vi "TrendsD01.vi"() -> ()   [LabVIEW 2019, in "D01.lvlib"]
uses:
  D01.lvlib
  <vilib>/measure/mamon.llb/Trigger Detection for 1 Channel.vi
  <vilib>/measure/NI_MAPro.lvlib
panel:
  out "No Change":bool
  out "Sudden Change":bool
  out "Decrease":bool
  out "Increase":bool
  out "Previous  ES":dbl
  out "Present  Speed":dbl
  out "Present Error":dbl format="%#.2g"
  out "Previous Error":dbl
  out "Previous  Speed":dbl
  out "Previous PW":dbl caption="Control Information"
  out "Pulse Trends":waveform(i16)[](graph) caption="Waveform Chart - Dark"
  in  "Close":bool
  out "disc name":string="Disc 01 Trends"
  out "dsgs":string="DSGS"
  out "Speed Trend":waveform(dbl)(graph) caption="Waveform Chart - Dark"
  out "Average Trend":waveform(dbl)[](graph) caption="Waveform Chart - Dark"
  out "Live Trend":waveform(dbl)[](graph) caption="Waveform Chart - Dark"
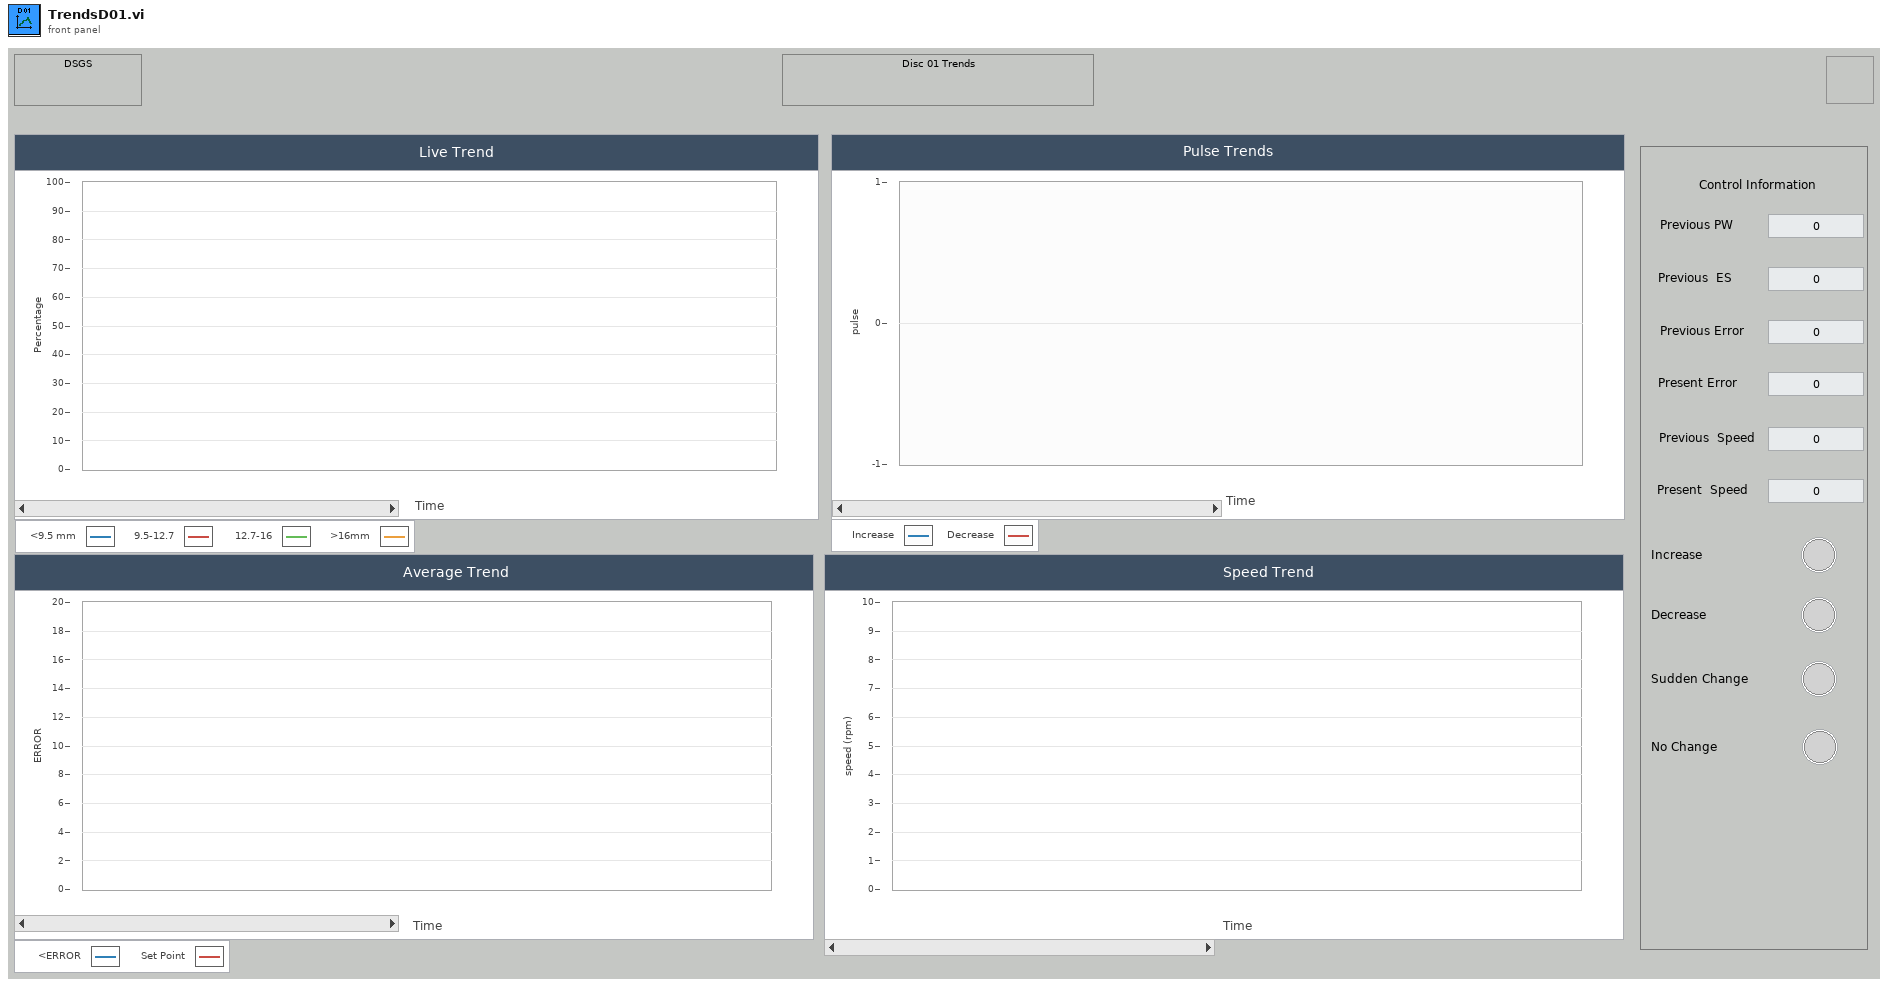
[diagram p1: front panel]
types:
  T1 = cluster{"decrease D01":bool, "increase D01":bool, "no change D01":bool, "sudden change D01":bool, "last error 01":dbl, "previous speed D01":dbl, "puls width D01":dbl, "slope D01":dbl}
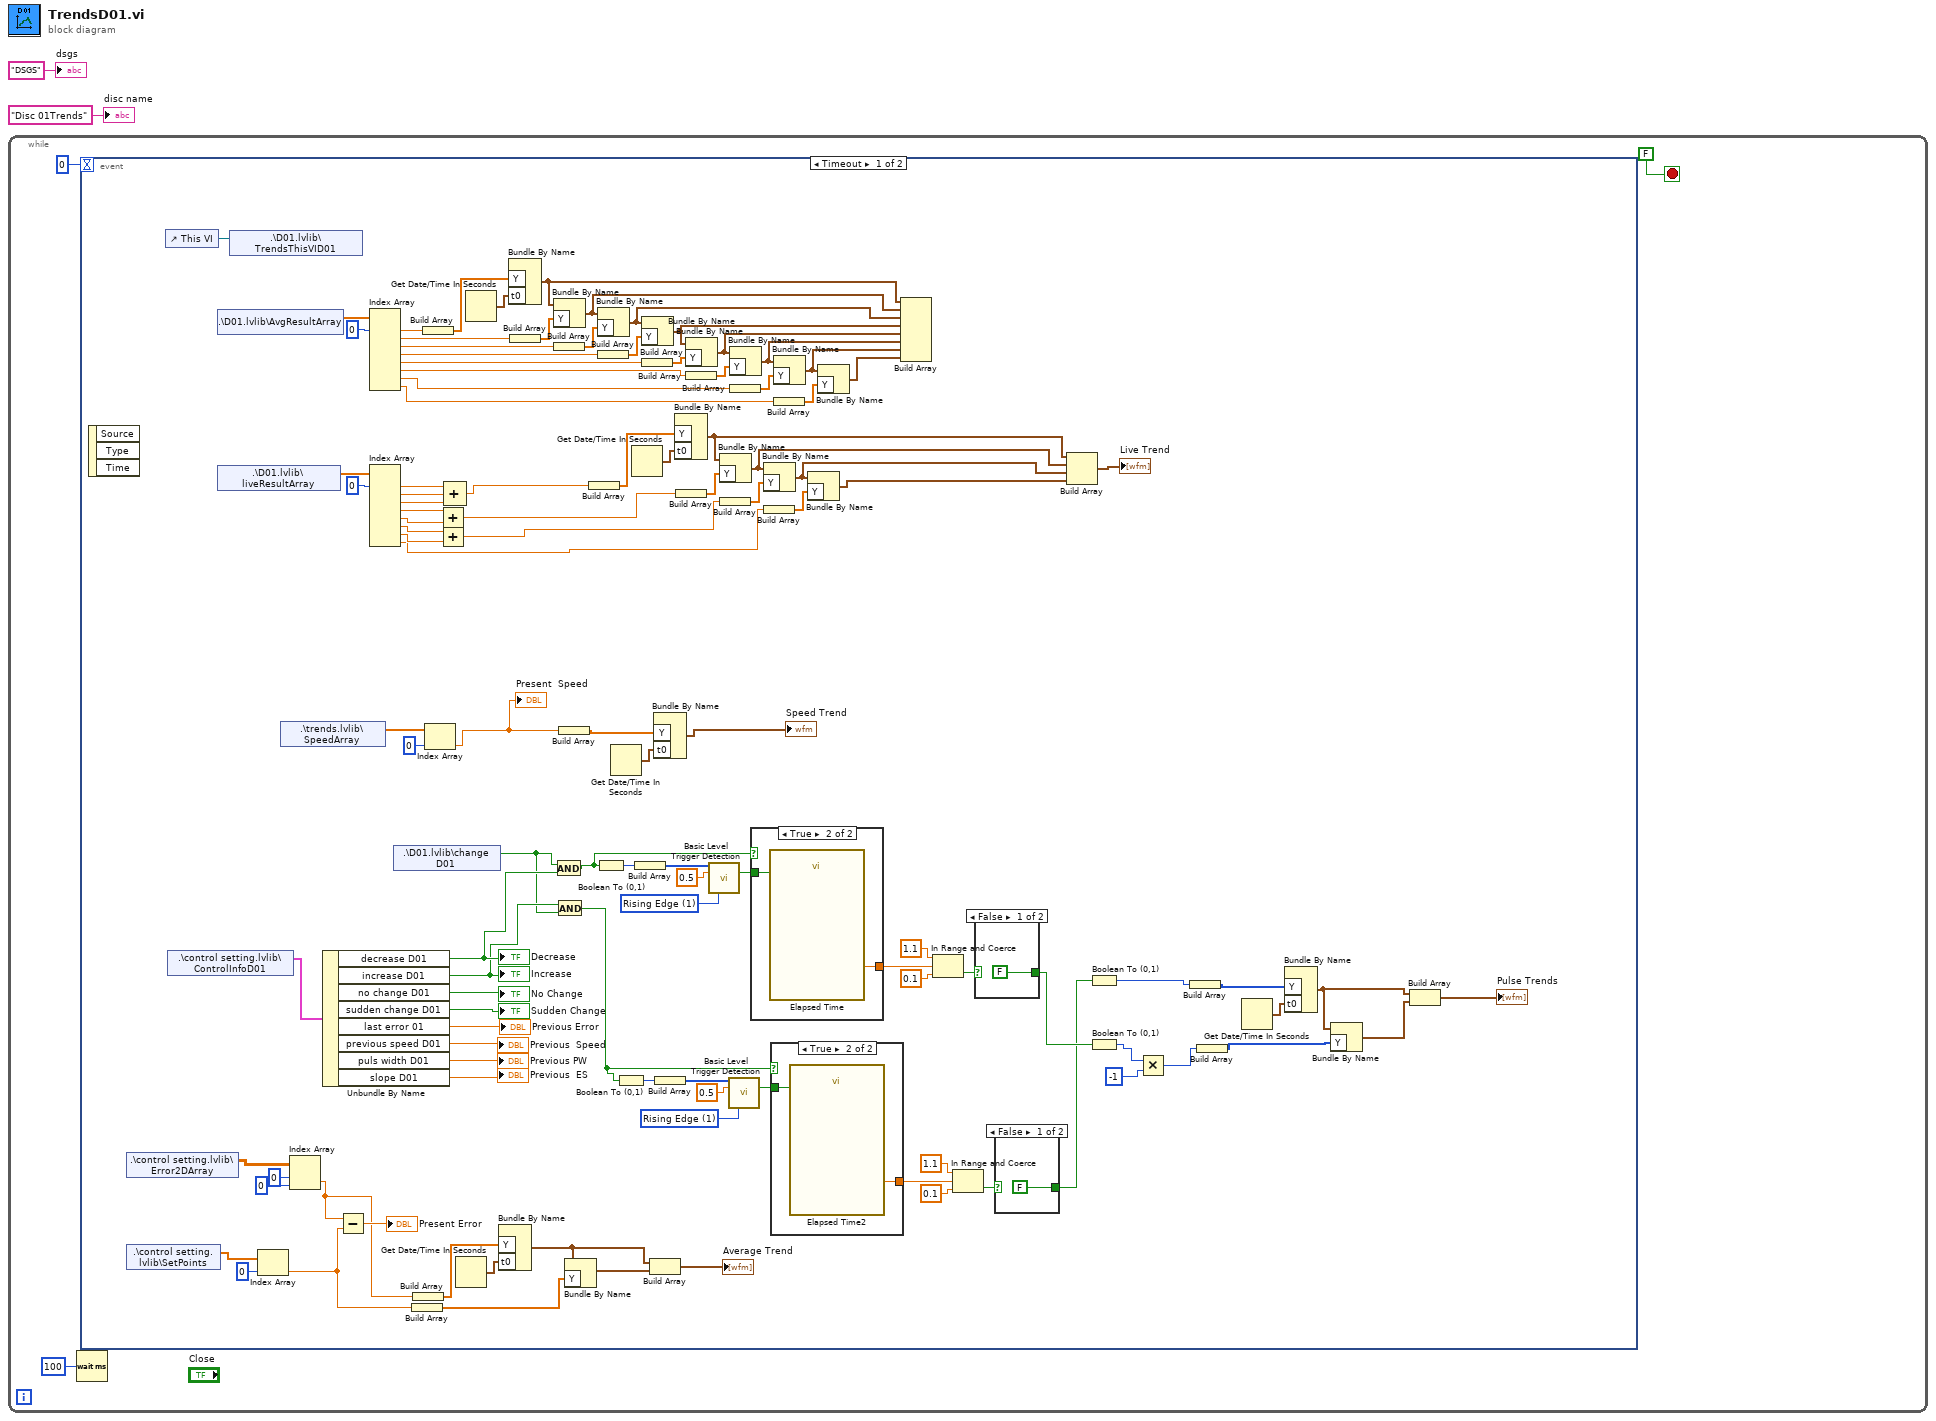
[diagram p0: block diagram]
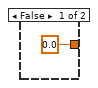
[diagram p3: hidden frame]
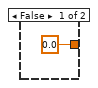
[diagram p5: hidden frame]
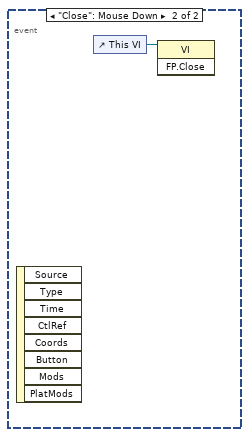
[diagram p6: hidden frame]
diagram:
  n1 = while {
    stop <- FALSE stop-if-true
    n2 = Wait (ms)(milliseconds to wait=u32 100) -> ()  [unwired: 1 out]
    n3 = event shown="[0] Timeout" {
      selector: _ -> [_ _]
      dyn-events: _ -> [_ _]
      timeout: 0 -> [_ _]
      event Timeout {
        w37 = u16 1 items=["Falling Edge", "Rising Edge"] ("trigger slope")
        w40 = u16 1 items=["Falling Edge", "Rising Edge"] ("trigger slope")
        n4 = event-data() -> ()  [unwired: 1 in, 3 out]
        n5 = shared-variable ".\\control setting.lvlib\\Error2DArray"() -> (w23:dbl[][])  [unwired: 1 in, 1 out]
        n6 = shared-variable ".\\control setting.lvlib\\SetPoints"() -> (w55:dbl[])  [unwired: 1 in, 1 out]
        n7 = control-ref of="This VI"() -> (w79:refnum<vi>)
        n8 = shared-variable ".\\control setting.lvlib\\ControlInfoD01"() -> (w63:T1)  [unwired: 1 in, 1 out]
        n9 = shared-variable ".\\D01.lvlib\\AvgResultArray"() -> (w85:dbl[])  [unwired: 1 in, 1 out]
        n10 = shared-variable ".\\D01.lvlib\\liveResultArray"() -> (w118:dbl[])  [unwired: 1 in, 1 out]
        n11 = shared-variable ".\\D01.lvlib\\TrendsThisVID01"(w79) -> ()  [unwired: 1 in, 1 out]
        n12 = Index Array(array=w55, index=0) -> (element=w11:dbl)
        n13 = shared-variable ".\\trends.lvlib\\SpeedArray"() -> (w68:dbl[])  [unwired: 1 in, 1 out]
        n14 = Index Array(array=w23, index (row)=0, index (col)=0 ("disabled index (col)")) -> (element=w6:dbl)
        n15 = Unbundle By Name(w63) -> ("decrease D01"=w51:bool, "increase D01"=w50:bool, "no change D01"=→"No Change":bool, "sudden change D01"=→"Sudden Change":bool, "last error 01"=→"Previous Error":dbl, "previous speed D01"=→"Previous  Speed":dbl, "puls width D01"=→"Previous PW":dbl, "slope D01"=→"Previous  ES":dbl)
        "Increase" <- w50
        "Decrease" <- w51
        n16 = Subtract(x=w6, y=w11) -> (x-y=→"Present Error":dbl)
        n17 = Index Array(array=w85, index #1=0 ("index")) -> (element #1=w95:dbl, element #2=w96:dbl, element #3=w98:dbl, element #4=w100:dbl, element #5=w101:dbl, element #6=w103:dbl, element #7=w105:dbl, element #8=w84:dbl)  [unwired: 7 in]
        n18 = Index Array(array=w118, index #1=0 ("index")) -> (element #1=w22:dbl, element #2=w21:dbl, element #3=w20:dbl, element #4=w18:dbl, element #5=w17:dbl, element #6=w16:dbl, element #7=w15:dbl, element #8=w12:dbl)  [unwired: 7 in]
        n19 = shared-variable ".\\D01.lvlib\\change D01"() -> (w49:bool)  [unwired: 1 in, 1 out]
        n20 = Build Array(w11) -> (w10:dbl[])
        n21 = Build Array(w6) -> (w26:dbl[])
        n22 = Build Array(w95) -> (w106:dbl[])
        n23 = Index Array(array=w68, index=0) -> (element=w52:dbl)
        "Present  Speed" <- w52
        n24 = Add(x=w18, y=w17) -> (x+y=w14:dbl)
        n25 = Add(x=w16, y=w15) -> (x+y=w13:dbl)
        n26 = Compound Arithmetic op=ADD(w22, w21, w20) -> (w19:dbl)
        n27 = Get Date/Time In Seconds() -> (seconds since 1Jan1904=w25:timestamp)
        n28 = Get Date/Time In Seconds() -> (seconds since 1Jan1904=w88:timestamp)
        n29 = Bundle By Name("Y"=w26, "t0"=w25) -> (w9:waveform(dbl))  [unwired: 1 in]
        n30 = Bundle By Name("Y"=w106, "t0"=w88) -> (w94:waveform(dbl))  [unwired: 1 in]
        n31 = Build Array(w96) -> (w97:dbl[])
        n32 = Bundle By Name(cluster=w94, "Y"=w97) -> (w93:waveform(dbl))
        n33 = Build Array(w98) -> (w99:dbl[])
        n34 = And(x=w49, y=w51) -> (x .and. y?=w39:bool)
        n35 = And(x=w50, y=w49) -> (x .and. y?=w27:bool)
        n36 = Build Array(w52) -> (w66:dbl[])
        n37 = Bundle By Name(cluster=w9, "Y"=w10) -> (w8:waveform(dbl))
        n38 = Build Array(w19) -> (w108:dbl[])
        n39 = Boolean To (0,1)(Boolean=w39) -> (0, 1=w48:i16)
        n40 = Bundle By Name(cluster=w93, "Y"=w99) -> (w92:waveform(dbl))
        n41 = Build Array(w100) -> (w87:dbl[])
        n42 = Get Date/Time In Seconds() -> (seconds since 1Jan1904=w65:timestamp)
        n43 = Boolean To (0,1)(Boolean=w27) -> (0, 1=w29:i16)
        n44 = Get Date/Time In Seconds() -> (seconds since 1Jan1904=w115:timestamp)
        n45 = Build Array(w48) -> (w47:i16[])
        n46 = Bundle By Name(cluster=w92, "Y"=w87) -> (w91:waveform(dbl))
        n47 = Build Array(w101) -> (w102:dbl[])
        n48 = Build Array(w9, w8) -> (→"Average Trend":waveform(dbl)[])
        n49 = Bundle By Name("Y"=w66, "t0"=w65) -> (→"Speed Trend":waveform(dbl))  [unwired: 1 in]
        n50 = Build Array(w29) -> (w30:i16[])
        n51 = Bundle By Name("Y"=w108, "t0"=w115) -> (w111:waveform(dbl))  [unwired: 1 in]
        n52 = Build Array(w14) -> (w110:dbl[])
        n53 = Bundle By Name(cluster=w91, "Y"=w102) -> (w90:waveform(dbl))
        n54 = Build Array(w103) -> (w104:dbl[])
        n55 = call-poly <vilib>:"Basic Level Trigger Detection.vi"("signal in"=w47, "level"=0.5, "trigger slope"=w40) -> ("trigger detected?"=w42:bool)  [unwired: 10 in, 2 out]
        n56 = Bundle By Name(cluster=w111, "Y"=w110) -> (w112:waveform(dbl))
        n57 = Build Array(w13) -> (w109:dbl[])
        n58 = call-poly <vilib>:"Basic Level Trigger Detection.vi"("signal in"=w30, "level"=0.5, "trigger slope"=w37) -> ("trigger detected?"=w35:bool)  [unwired: 10 in, 2 out]
        n59 = Bundle By Name(cluster=w90, "Y"=w104) -> (w89:waveform(dbl))
        n60 = Build Array(w105) -> (w107:dbl[])
        n61 = case shown="True" w39 {
          tunnel: [0.0 ("Elapsed Time (s)") w128] -> w45
          tunnel: w42 -> [_ w127]
          frame False {
          }
          frame True {
            n62 = call "Elapsed Time"("Reset"=w127) -> ("Elapsed Time (s)"=w128:dbl)  [unwired: 11 in, 7 out]
          }
        }
        n63 = Bundle By Name(cluster=w112, "Y"=w109) -> (w113:waveform(dbl))
        n64 = Build Array(w12) -> (w116:dbl[])
        n65 = case shown="True" w27 {
          tunnel: [0.0 ("Elapsed Time (s)") w123] -> w32
          tunnel: w35 -> [_ w122]
          frame False {
          }
          frame True {
            n66 = call "Elapsed Time2"("Reset"=w122) -> ("Elapsed Time (s)"=w123:dbl)  [unwired: 11 in, 7 out]
          }
        }
        n67 = Bundle By Name(cluster=w89, "Y"=w107) -> (w81:waveform(dbl))
        n68 = Build Array(w84) -> (w83:dbl[])
        n69 = Bundle By Name(cluster=w113, "Y"=w116) -> (w114:waveform(dbl))
        n70 = Bundle By Name(cluster=w81, "Y"=w83) -> (w82:waveform(dbl))
        n71 = Build Array(w94, w93, w92, w91, w90, w89, w81, w82) -> ()  [unwired: 1 out]
        n72 = In Range and Coerce(upper limit=1.1, x=w45, lower limit=0.1) -> (In Range?=w41:bool)  [unwired: 1 out]
        n73 = In Range and Coerce(upper limit=1.1, x=w32, lower limit=0.1) -> (In Range?=w36:bool)  [unwired: 1 out]
        n74 = case shown="False" w41 {
          selector: w41 -> [_ w125]
          tunnel: [FALSE w125] -> w38
          frame False {
          }
          frame True {
          }
        }
        n75 = case shown="False" w36 {
          selector: w36 -> [_ w120]
          tunnel: [FALSE w120] -> w28
          frame False {
          }
          frame True {
          }
        }
        n76 = Build Array(w111, w112, w113, w114) -> (→"Live Trend":waveform(dbl)[])
        n77 = Boolean To (0,1)(Boolean=w28) -> (0, 1=w76:i16)
        n78 = Boolean To (0,1)(Boolean=w38) -> (0, 1=w72:i16)
        n79 = Multiply(x=w72, y=i16 -1 ("0, 1")) -> (x*y=w70:i16)
        n80 = Build Array(w76) -> (w77:i16[])
        n81 = Build Array(w70) -> (w75:i16[])
        n82 = Get Date/Time In Seconds() -> (seconds since 1Jan1904=w78:timestamp)
        n83 = Bundle By Name("Y"=w77, "t0"=w78) -> (w74:waveform(i16))  [unwired: 1 in]
        n84 = Bundle By Name(cluster=w74, "Y"=w75) -> (w73:waveform(i16))
        n85 = Build Array(w74, w73) -> (→"Pulse Trends":waveform(i16)[])
      }
      event "Close": Mouse Down {
        n86 = event-data() -> ()  [unwired: 1 in, 8 out]
        n87 = control-ref of="This VI"() -> (w129:refnum<vi>)
        n88 = invoke class="VI" method="FP.Close"(reference=w129) -> ()  [unwired: 2 in, 3 out]
      }
    }
  }
  "dsgs" <- "DSGS" ("dsgs")
  "disc name" <- "Disc 01Trends" ("disc name")
